vi "MainGui-ErrorConfirm.vi"(8 "error in (no error)":errorcluster) -> (0 "error out":errorcluster)   [LabVIEW 2016]
uses:
  MainGui.Action.ctl
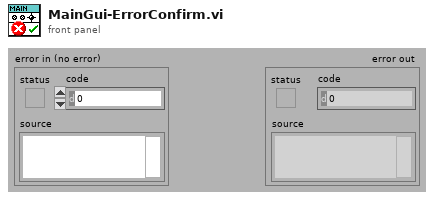
[diagram p1: front panel]
types:
  T1 = typedef "MainGui.Action.ctl" = enum32{"idle", "constructor", "destructor", "--- MainGui ---", "Gui.Resize", "Gui.Translate", "Error.Update", "Error.Confirm", "TopBar.Update", "Buttons.Update", "StatusMsg.Update", "StatusTable.Update", "LogsTable.Update", "ProductList.Update", "ProductTable.Update", "SetupVariantTable.Update"}
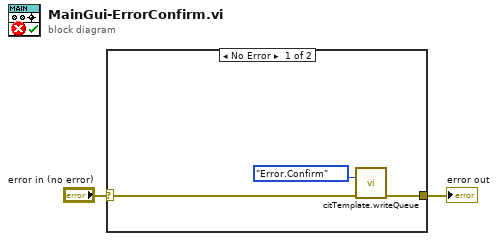
[diagram p0: block diagram]
diagram:
  n1 = case shown="No Error" "error in (no error)" {
    selector: "error in (no error)" -> [w3 w6]
    tunnel: [w5 w6] -> w1
    frame No Error {
      n2 = call "citTemplate.writeQueue.vi"("event in (if not connected:all statemachine with data event)"=MainGui.Action."Error.Confirm" ("Action"), "error in (no error)"=w3) -> ("error out"=w5:errorcluster)  [unwired: 13 in]
    }
    frame Error {
    }
  }
  "error out" <- w1
